vi "AverageFilter_Example.vi"() -> ()   [LabVIEW 2019]
uses:
  <vilib>/Rock Robotics/WPI/ThirdParty/JAS_Junk/TrajLib/MathUtil_Clamp.vi
  <vilib>/Rock Robotics/WPI/ThirdParty/JAS_Junk/TrajLib/LinearFilter_ResetToValue.vi
  <vilib>/Rock Robotics/WPI/ThirdParty/JAS_Junk/TrajLib/LinearFilter_Calculate.vi
  <vilib>/Rock Robotics/WPI/ThirdParty/JAS_Junk/TrajLib/LinearFilter_MovingAverage.vi
  <vilib>/Rock Robotics/WPI/ThirdParty/JAS_Junk/TrajLib/LinearFilter_LowPassBW1.vi
  <vilib>/Rock Robotics/WPI/ThirdParty/JAS_Junk/TrajLib/LinearFilter_LowPassBW2.vi
  <vilib>/Rock Robotics/WPI/ThirdParty/JAS_Junk/TrajLib/LinearFilter_HighPassBW1.vi
  <vilib>/Rock Robotics/WPI/ThirdParty/JAS_Junk/TrajLib/LinearFilter_HighPassBW2.vi
  <vilib>/Rock Robotics/WPI/ThirdParty/JAS_Junk/TrajLib/Trajectory_Library.lvlib
panel:
  in  "Auto / Manual\nProcess Variable\nGeneration":bool=TRUE
  in  "Enable\nNoise":bool=TRUE
  in  "Filter Enable":bool=TRUE
  in  "Use White Noise":bool=TRUE
  in  "Tab Control 2":enum32{"Avg 3", "Avg 7"}(tab)
  out "Avg3":cluster{dbl, dbl, "Value_Output":dbl}(graph)
  out "Avg3 Out Dial":dbl(knob)=-2.895988890827539e-05 scale=-20.0..20.0
  out "Avg3 Out":dbl format="%11.3f"
  out "Avg7":cluster{dbl, dbl, "Value_Output":dbl}(graph)
  out "Avg7 Out":dbl format="%11.3f"
  out "Avg7 Out Dial":dbl(knob)=-2.895988890827539e-05 scale=-20.0..20.0
  out "Loop Adjust":dbl format="%11.3f"
  in  "Manual\nInput":dbl(slide) min=-12.0 max=12.0 scale=-12.0..12.0
  out "Raw Noise":dbl(knob)=-2.895988890827539e-05 scale=-20.0..20.0
  out "Raw Noise":dbl format="%11.3f"
  out "Actual Input":dbl(knob)=-2.895988890827539e-05 scale=-20.0..20.0
  out "Actual Input":dbl format="%11.3f"
  out "Input":cluster{"Manual\nInput":dbl, dbl, "f":dbl}(graph)
  out "Meas Dial":dbl(knob)=-2.895988890827539e-05 scale=-20.0..20.0
  out "Measured Value":dbl format="%11.3f"
  # "Average Filter Example"
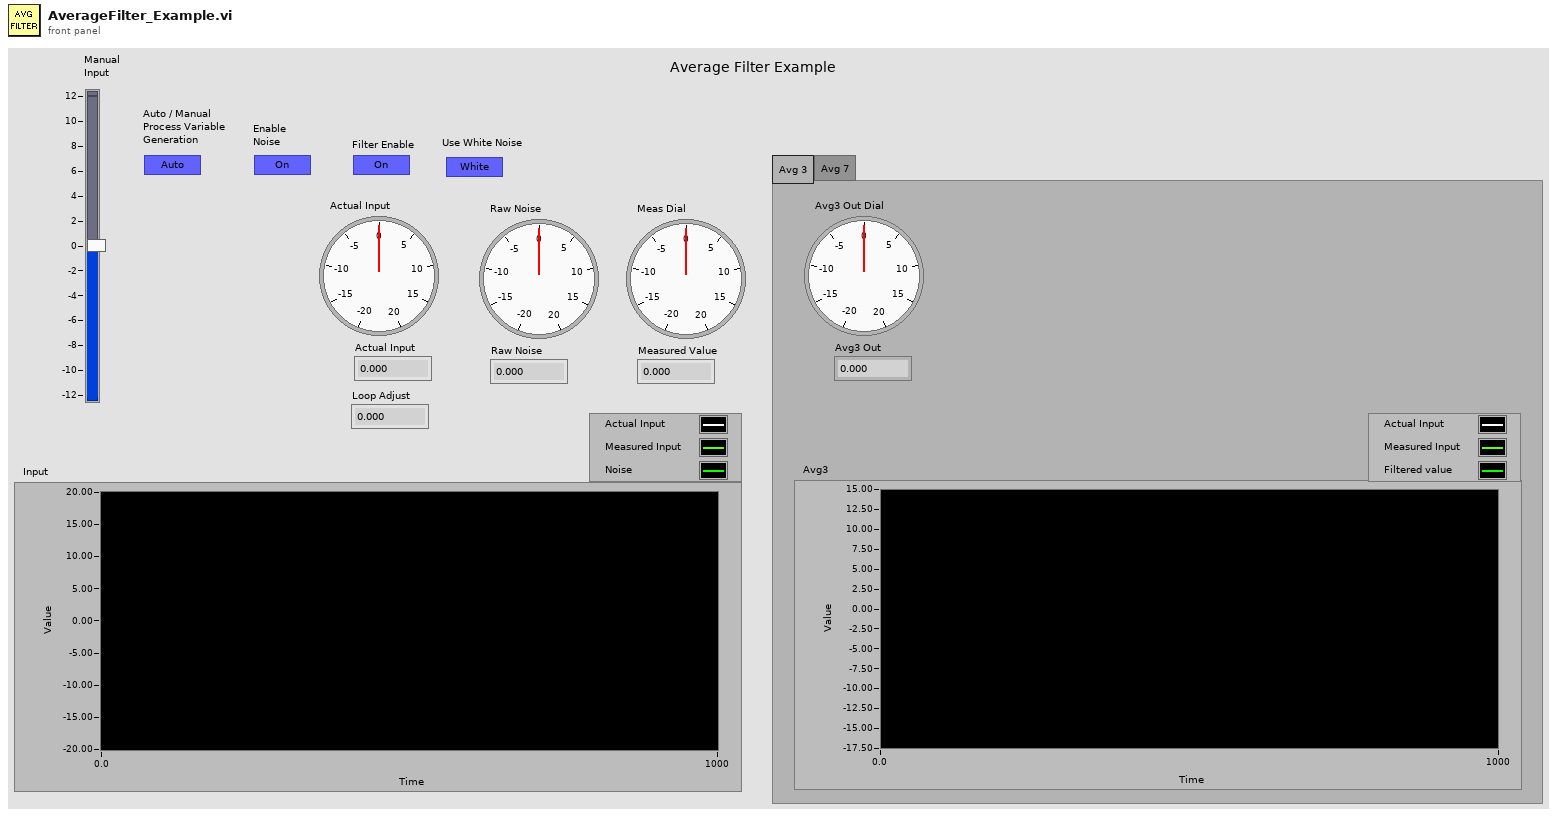
[diagram p1: front panel]
types:
  T1 = enum16{"Moving Average", "Low Pass 1st Order Butterworth", "Low Pass 2nd Order Butterworth", "High Pass 1st Order Butterworth", "High Pass 2nd Order Butterworth"}
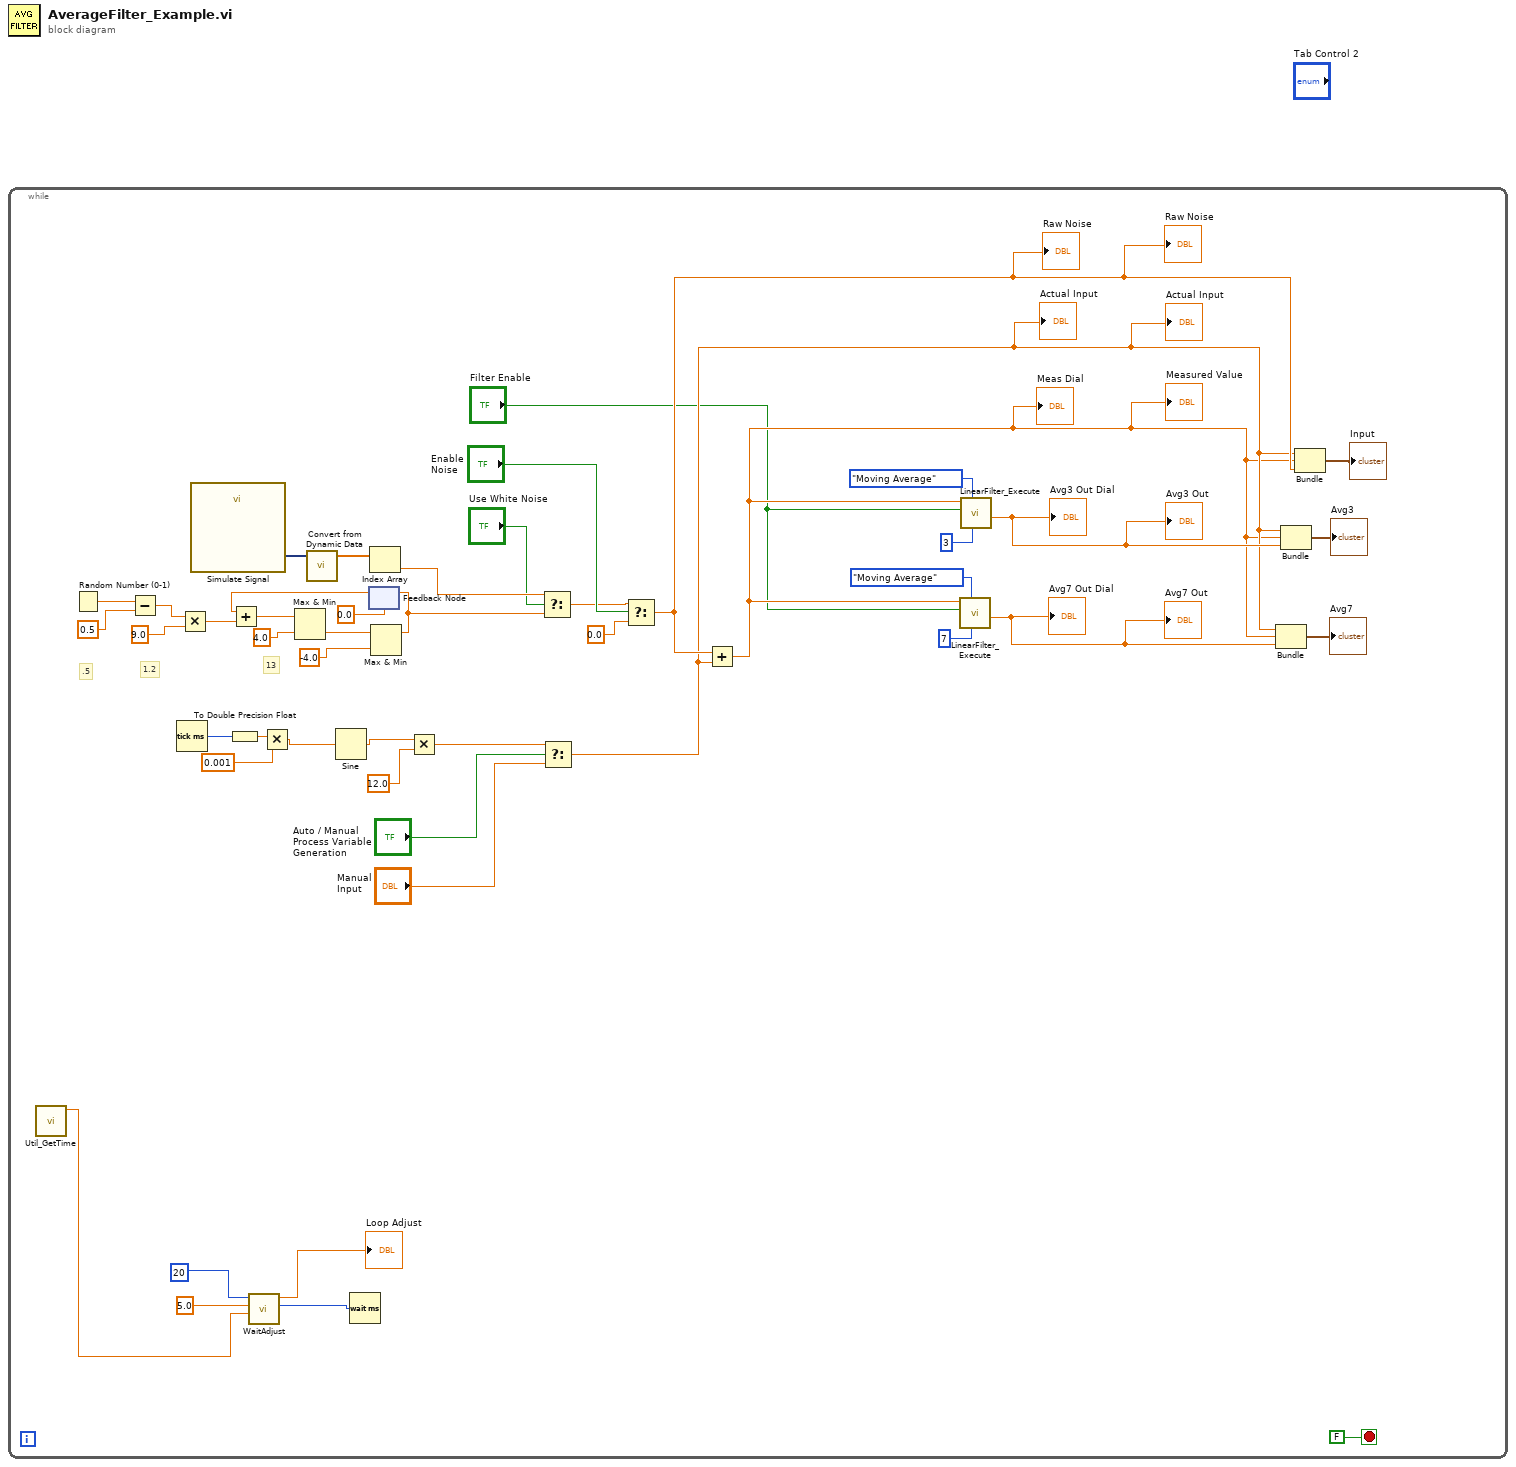
[diagram p0: block diagram]
diagram:
  n1 = while {
    stop <- FALSE stop-if-true
    # "13"
    # "1.2"
    # ".5"
    n2 = call <vilib>:"Util_GetTime.vi"() -> ("FPGA_Time_Seconds"=w2:dbl)  [unwired: 10 in, 1 out]
    n3 = Random Number (0-1)() -> (number: 0 to 1=w42:dbl)
    n4 = Subtract(x=w42, y=0.5) -> (x-y=w38:dbl)
    n5 = Tick Count (ms)() -> (millisecond timer value=w33:u32)
    n6 = Multiply(x=w38, y=9.0) -> (x*y=w37:dbl)
    n7 = call "Simulate Signal"() -> ("DC with Uniform Noise"=w21:dynamicdata)  [unwired: 14 in, 1 out]
    n8 = To Double Precision Float(number=w33) -> (double precision float=w34:dbl)
    n9 = call <vilib>:"WaitAdjust.vi"("Time_SEC"=w2, "MaxDeviation_MS"=5.0, "DesiredLoopTime_MS"=u32 20 ("milliseconds to wait")) -> ("AdjustedWaitTime_MS"=w4:u32, "Offset_MS"=→"Loop Adjust":dbl)  [unwired: 7 in]
    n10 = Multiply(x=w34, y=0.001) -> (x*y=w31:dbl)
    n11 = call "Convert from Dynamic Data"("Dynamic Data Type"=w21) -> ("Array"=w20:dbl[])  [unwired: 3 in]
    n12 = Sine(x=w31) -> (sin(x)=w30:dbl)
    n13 = Wait (ms)(milliseconds to wait=w4) -> ()  [unwired: 1 out]
    n14 = feedback #1(0.0) -> (w39:dbl)
    n15 = Add(x=w39, y=w37) -> (x+y=w41:dbl)
    n16 = Max & Min(x=w41, y=4.0) -> (min(x,y)=w40:dbl)  [unwired: 1 out]
    n17 = Index Array(array=w20) -> (element=w19:dbl)  [unwired: 1 in]
    n18 = Max & Min(x=w40, y=-4.0) -> (max(x,y)=w22:dbl)  [unwired: 1 out]
    n19 = feedback-in #1(w22) -> ()
    n20 = Multiply(x=w30, y=12.0) -> (x*y=w27:dbl)
    n21 = Select(t=w19, s="Use White Noise", f=w22) -> (s? t:f=w23:dbl)
    n22 = Select(t=w27, s="Auto / Manual\nProcess Variable\nGeneration", f="Manual\nInput") -> (s? t:f=w8:dbl)
    "Actual Input" <- w8
    "Actual Input" <- w8
    n23 = Select(t=w23, s="Enable\nNoise", f=0.0) -> (s? t:f=w17:dbl)
    "Raw Noise" <- w17
    "Raw Noise" <- w17
    n24 = Add(x=w17, y=w8) -> (x+y=w7:dbl)
    "Measured Value" <- w7
    "Meas Dial" <- w7
    n25 = call <vilib>:"LinearFilter_Execute.vi"("Samples"=7, "Filter Type"=T1."Moving Average", "Enable"="Filter Enable", "Input"=w7) -> ("Output"=w14:dbl)  [unwired: 6 in, 1 out]
    "Avg7 Out" <- w14
    "Avg7 Out Dial" <- w14
    n26 = call <vilib>:"LinearFilter_Execute.vi"("Samples"=3, "Filter Type"=T1."Moving Average", "Enable"="Filter Enable", "Input"=w7) -> ("Output"=w15:dbl)  [unwired: 6 in, 1 out]
    "Avg3 Out" <- w15
    "Avg3 Out Dial" <- w15
    n27 = Bundle("Manual\nInput"=w8, w7, "Output"=w14) -> (→"Avg7":cluster{"Manual\nInput":dbl, dbl, "Output":dbl})  [unwired: 1 in]
    n28 = Bundle("Manual\nInput"=w8, w7, "Output"=w15) -> (→"Avg3":cluster{"Manual\nInput":dbl, dbl, "Output":dbl})  [unwired: 1 in]
    n29 = Bundle("Manual\nInput"=w8, w7, "f"=w17) -> (→"Input":cluster{"Manual\nInput":dbl, dbl, "f":dbl})  [unwired: 1 in]
  }
